vi "SetAutoArmedRoutines.vi"(1 "Routine_RRR":string, 2 "Routine_RLR":string, 3 "Routine_LRL":string, 4 "Routine_LLL":string) -> ()   [LabVIEW 2017]
uses:
  <vilib>/Rock Robotics/Network Tables/NT Write String.vi
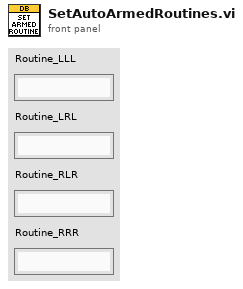
[diagram p1: front panel]
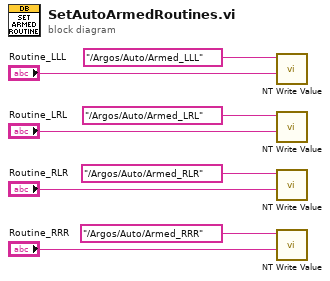
[diagram p0: block diagram]
diagram:
  n1 = call-poly <vilib>:"NT Write Value.vi"("String"="Routine_LLL", "Name"="/Argos/Auto/Armed_LLL") -> ()  [unwired: 9 in, 1 out]
  n2 = call-poly <vilib>:"NT Write Value.vi"("String"="Routine_LRL", "Name"="/Argos/Auto/Armed_LRL") -> ()  [unwired: 9 in, 1 out]
  n3 = call-poly <vilib>:"NT Write Value.vi"("String"="Routine_RLR", "Name"="/Argos/Auto/Armed_RLR") -> ()  [unwired: 9 in, 1 out]
  n4 = call-poly <vilib>:"NT Write Value.vi"("String"="Routine_RRR", "Name"="/Argos/Auto/Armed_RRR") -> ()  [unwired: 9 in, 1 out]
